vi "handle error.vi"(0 "Serial port assistant model in":refnum<class "Serial port assistant model.lvclass">, 11 "error in (no error)":errorcluster) -> (4 "Serial port assistant model out":refnum<class "Serial port assistant model.lvclass">, 15 "error out":errorcluster)   [LabVIEW 2022 SP3, in "Serial port assistant model.lvlib" / "Serial port assistant model.lvclass"]
uses:
  Serial port assistant model.lvclass
  Serial port assistant model.lvclass/Serial port assistant model.ctl
  changed data--type.ctl
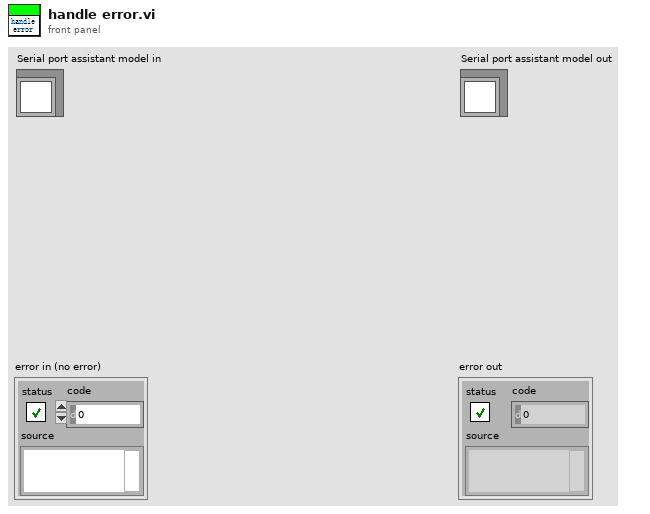
[diagram p1: front panel]
types:
  T1 = cluster{"changed data":string, "status":bool, "code":i32, "source":string}
  T2 = typedef "Serial port assistant model.lvlib/Serial port assistant model.lvclass/changed data--type.ctl" = cluster{"changed data":string}
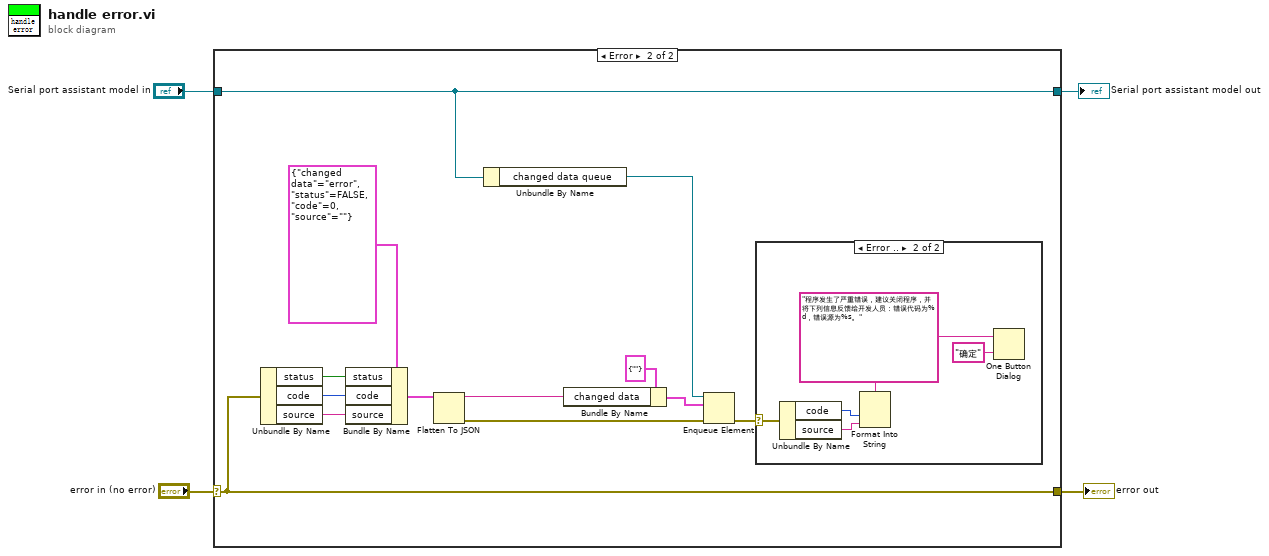
[diagram p0: block diagram]
diagram:
  n1 = case shown="Error" "error in (no error)" {
    selector: "error in (no error)" -> [w5 w9]
    tunnel: [w5 w9] -> w3
    tunnel: [w6 w8] -> w1
    tunnel: "Serial port assistant model in" -> [w6 w8]
    frame No Error {
    }
    frame Error {
      n2 = Unbundle By Name(w9) -> ("status"=w14:bool, "code"=w13:i32, "source"=w12:string)
      n3 = Bundle By Name(cluster=T1 {"changed data"="error", "status"=FALSE, "code"=0, "source"=""}, "status"=w14, "code"=w13, "source"=w12) -> (w11:T1)
      n4 = Flatten To JSON(anything=w11) -> (JSON string=w10:string, 11:w16:errorcluster)  [unwired: 2 in]
      n5 = Unbundle By Name(w8) -> ("changed data queue"=w19:refnum<queue>)
      n6 = Bundle By Name(cluster=T2 {"changed data"=""} ("element"), "changed data"=w10) -> (w17:T2)
      n7 = Enqueue Element(queue=w19, element=w17, error in (no error)=w16) -> (error out=w7:errorcluster)  [unwired: 1 in, 2 out]
      n8 = case shown="Error .." w7 {
        selector: w7 -> [_ w24]
        frame No Error {
        }
        frame Error {
          w21 = "程序发生了严重错误，建议关闭程序，并将下列信息反馈给开发人员：错误代码为%d，错误源为%s。" ("format string")
          n9 = Unbundle By Name(w24) -> ("code"=w23:i32, "source"=w22:string)
          n10 = Format Into String(format string=w21, w23, w22) -> ()  [unwired: 2 in, 2 out]
          n11 = One Button Dialog(message=w21, button name ("OK")="确定") -> ()  [unwired: 1 out]
        }
      }
    }
  }
  "error out" <- w3
  "Serial port assistant model out" <- w1
